vi "stringracer.vi"() -> ()   [LabVIEW 2021]
panel:
  out "orig string racer":string
  out "string racer jf2":string
  in  "It's wonderfull! Don't STOP it!":bool
  out "string racer jf1":string
  in  "enter your string, please":string
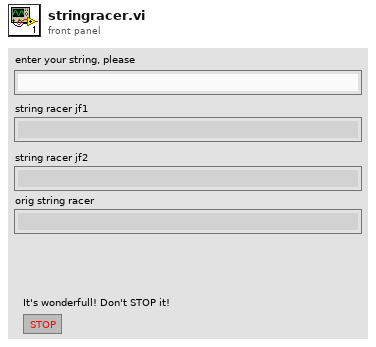
[diagram p1: front panel]
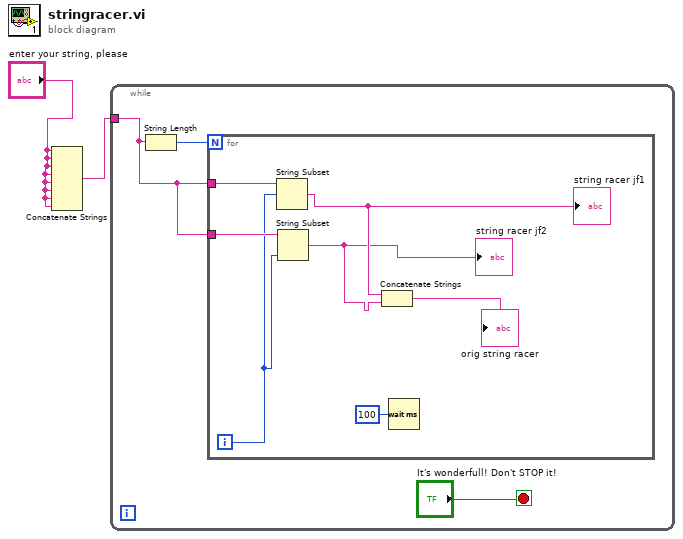
[diagram p0: block diagram]
diagram:
  n1 = Concatenate Strings("enter your string, please", "enter your string, please", "enter your string, please", "enter your string, please", "enter your string, please", "enter your string, please", "enter your string, please", "enter your string, please") -> (w1:string)
  n2 = while {
    tunnel: w1 -> [w3]
    stop <- "It's wonderfull! Don't STOP it!" stop-if-true
    n3 = String Length(string=w3) -> (length=w5:i32)
    n4 = for {
      N: w5 -> [_]
      tunnel: w3 -> [w12]
      tunnel: w3 -> [w10]
      i -> [w9]
      n5 = String Subset(string=w12, offset (0)=w9) -> (substring=w8:string)  [unwired: 1 in]
      "string racer jf1" <- w8
      n6 = String Subset(string=w10, length (rest)=w9) -> (substring=w6:string)  [unwired: 1 in]
      "string racer jf2" <- w6
      n7 = Concatenate Strings(w8, w6) -> (→"orig string racer":string)
      n8 = Wait (ms)(milliseconds to wait=u32 100) -> ()  [unwired: 1 out]
    }
  }
